vi "Delete Annotation.vi"(8 "error in (no error)":errorcluster, 10 "Name":string, 11 "FSM.Edge in":refnum<class "FSM.Edge.lvclass">) -> (0 "error out":errorcluster, 2 "Changed?":bool, 3 "FSM.Edge out":refnum<class "FSM.Edge.lvclass">)   [LabVIEW 2015, in "FSM.Edge.lvclass"]
uses:
  FSM.Edge.lvclass
  FSM.Edge.lvclass/FSM.Edge.ctl
  FSM.Annotation/FSM.Annotation.lvclass
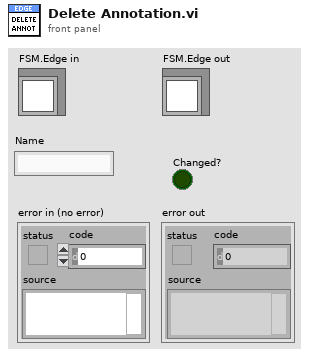
[diagram p1: front panel]
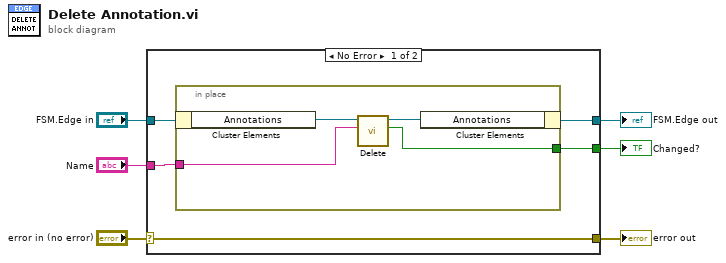
[diagram p0: block diagram]
diagram:
  n1 = case shown="No Error" "error in (no error)" {
    selector: "error in (no error)" -> [w11 w17]
    tunnel: [w11 w17] -> w5
    tunnel: [w8 w16] -> w4
    tunnel: "Name" -> [w10 _]
    tunnel: "FSM.Edge in" -> [w9 w16]
    tunnel: [w7 _] -> w1
    frame No Error {
      n2 = in-place {
        in-place-border: w10 -> [w13]
        in-place-border: [w12] -> w7
        n3 = in-place-cluster #1(w9) -> ("Annotations"=w15:refnum<class "FSM.Annotation.lvclass">)
        n4 = call "Delete.vi"("Name"=w13, "FSM.Annotation in"=w15) -> ("Changed?"=w12:bool, "FSM.Annotation out"=w14:refnum<class "FSM.Annotation.lvclass">)  [unwired: 7 in, 1 out]
        n5 = in-place-cluster #1("Annotations"=w14) -> (w8:refnum<class "FSM.Edge.lvclass">)
      }
    }
    frame Error {
    }
  }
  "error out" <- w5
  "FSM.Edge out" <- w4
  "Changed?" <- w1
